vi "Varient_number_check.vi"(8 "error in":errorcluster, 10 "Varient path":path, 11 "Varient No.":u16) -> (0 "error out":errorcluster, 1 "Batch Size":i32, 2 "Varient Number":i32, 3 "Part Name":string, 4 "PART_NO":string, 5 "TORISHI_CODE":string, 6 "MODEL LIST":string[](array[string]))   [LabVIEW 2017]
uses:
  <vilib>/Utility/config.llb/Read Key (I32).vi
  <vilib>/Utility/config.llb/Read Key (String).vi
  <vilib>/Utility/config.llb/NI_LVConfig.lvlib
panel:
  # "Varient no. check"
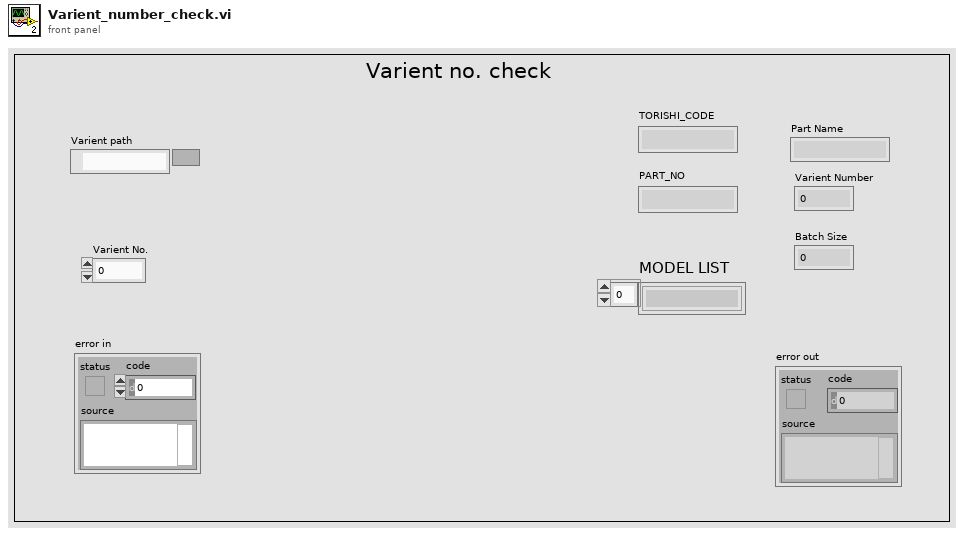
[diagram p1: front panel]
types:
  T1 = typedef "NI_LVConfig.lvlib/Config Data RefNum.ctl" = refnum<k1>
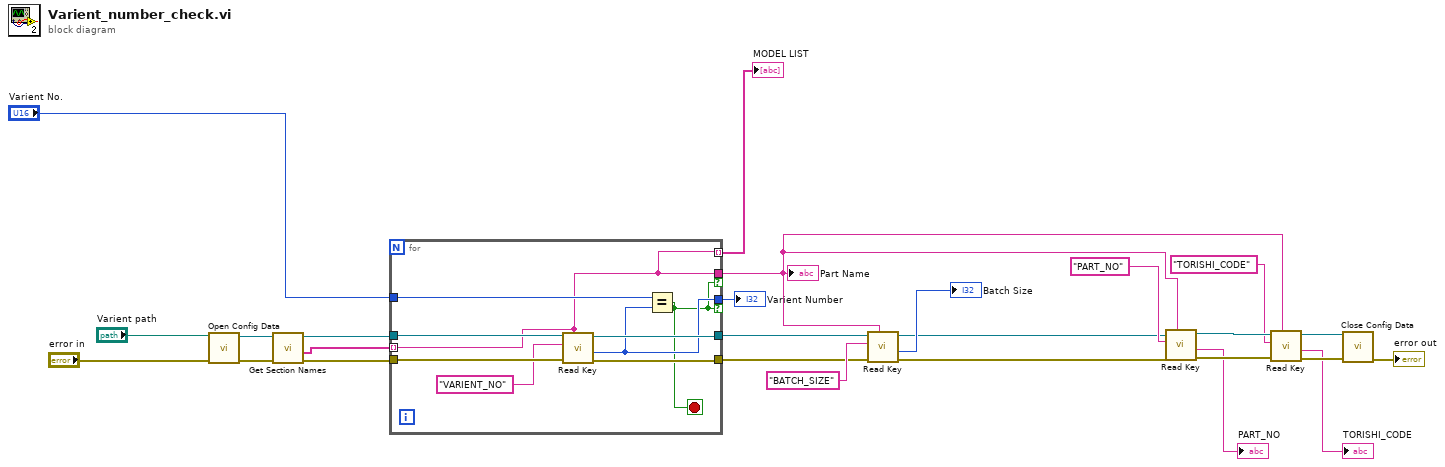
[diagram p0: block diagram]
diagram:
  n1 = call <vilib>:"Open Config Data.vi"("error in (no error)"="error in", "configuration file path"="Varient path") -> ("error out"=w25:errorcluster, "refnum"=w26:T1)  [unwired: 7 in, 1 out]
  n2 = call <vilib>:"Get Section Names.vi"("error in (no error)"=w25, "refnum"=w26) -> ("error out"=w23:errorcluster, "section names"=w21:string[], "refnum out"=w22:T1)  [unwired: 7 in]
  n3 = for {
    tunnel: w21 -> [w27] mode=indexing
    tunnel: w22 -> [w33]
    tunnel: [w32] -> w16
    tunnel: w23 -> [w35]
    tunnel: [w34] -> w17
    tunnel: [w29] -> w19 if=w28
    tunnel: "Varient No." -> [w30]
    tunnel: [w27] -> w6 if=w28
    tunnel: [w27] -> w1 mode=indexing
    stop <- w28 stop-if-true
    n4 = call-poly <vilib>:"Read Key.vi"("section"=w27, "error in (no error)"=w35, "key"="VARIENT_NO" ("name or relative path"), "refnum"=w33) -> ("error out"=w34:errorcluster, "value"=w29:i32, "refnum out"=w32:T1)  [unwired: 4 in, 1 out]
    n5 = Equal?(x=w30, y=w29) -> (x = y?=w28:bool)
  }
  "Varient Number" <- w19
  "Part Name" <- w6
  "MODEL LIST" <- w1
  n6 = call-poly <vilib>:"Read Key.vi"("section"=w6, "error in (no error)"=w17, "key"="BATCH_SIZE" ("name or relative path"), "refnum"=w16) -> ("error out"=w8:errorcluster, "value"=→"Batch Size":i32, "refnum out"=w10:T1)  [unwired: 4 in, 1 out]
  n7 = call-poly <vilib>:"Read Key.vi"("section"=w6, "error in (no error)"=w8, "key"="PART_NO", "refnum"=w10) -> ("error out"=w13:errorcluster, "value"=→"PART_NO":string, "refnum out"=w14:T1)  [unwired: 4 in, 1 out]
  n8 = call-poly <vilib>:"Read Key.vi"("section"=w6, "error in (no error)"=w13, "key"="TORISHI_CODE", "refnum"=w14) -> ("error out"=w7:errorcluster, "value"=→"TORISHI_CODE":string, "refnum out"=w9:T1)  [unwired: 4 in, 1 out]
  n9 = call <vilib>:"Close Config Data.vi"("error in (no error)"=w7, "refnum"=w9) -> ("error out"=→"error out":errorcluster)  [unwired: 8 in, 1 out]
